vi "g_timeout.vi"() -> ()   [LabVIEW 2023]
panel:
  in  "g_timeout":i32=-1
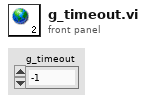
[diagram p1: front panel]
diagram:
